vi "Wait For LACK OF Front Panel Activity.vi"(1 "Delay (ms)":i32=1000, 2 "Generic VI Reference":refnum<vi>) -> ()   [LabVIEW 2013]
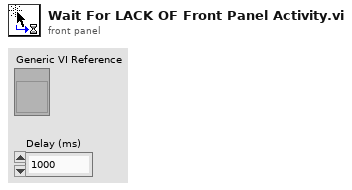
[diagram p1: front panel]
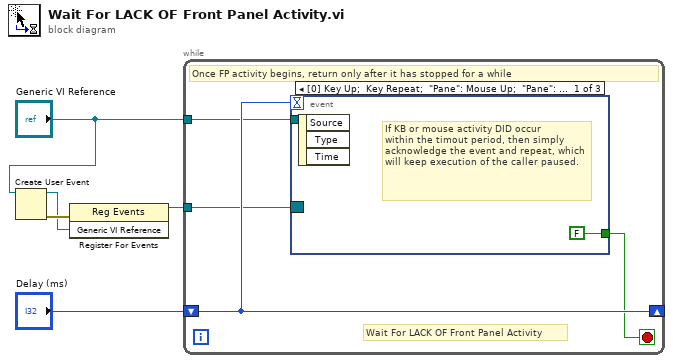
[diagram p0: block diagram]
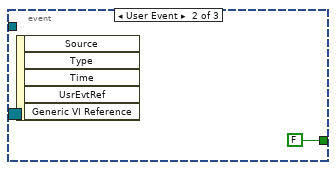
[diagram p2: hidden frame]
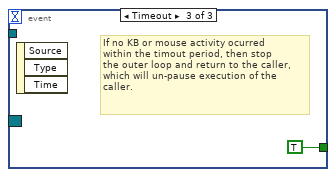
[diagram p3: hidden frame]
diagram:
  n1 = Create User Event(user event datatype="Generic VI Reference") -> (user event=w2:refnum<user-event>, error out=w3:errorcluster)  [unwired: 1 in]
  n2 = register-events(error in=w3, w2) -> (reference out=w4:refnum<event-registration>)  [unwired: 1 in, 1 out]
  n3 = while {
    shift-right: [w9] -> _
    shift-left: "Delay (ms)" -> [w9]
    tunnel: w4 -> [w7]
    tunnel: "Generic VI Reference" -> [w6]
    stop <- w8 stop-if-true
    # "Wait For LACK OF Front Panel Activity"
    # "Once FP activity begins, return only after it has stopped for a while"
    n4 = event shown="[0] Key Up;  Key Repeat;  \"Pane\": Mouse Up;  \"Pane\": Mouse Move;  \"Pane\": Mouse Wheel;  \"Pane\": Mouse Enter;  Key Down" {
      selector: w7 -> [_ _ _]
      dyn-events: _ -> [_ _ _]
      timeout: w9 -> [_ _ _]
      tunnel: [FALSE FALSE TRUE] -> w8
      tunnel: w6 -> [_ _ _]
      event Key Up; Key Repeat; Mouse Up; Mouse Move; Mouse Wheel; Mouse Enter; Key Down {
        # "If KB or mouse activity DID occur\nwithin the timout period, then simply acknowledge the event and repeat, which will keep execution of the caller paused."
        n5 = event-data() -> ()  [unwired: 1 in, 3 out]
      }
      event User Event {
        n6 = event-data() -> ()  [unwired: 1 in, 5 out]
      }
      event Timeout {
        # "If no KB or mouse activity ocurred \nwithin the timout period, then stop \nthe outer loop and return to the caller, which will un-pause execution of the caller."
        n7 = event-data() -> ()  [unwired: 1 in, 3 out]
      }
    }
  }
